vi "Coll_Det_Example.vi"() -> ()   [LabVIEW 2011]
uses:
  SObject.ctl
  Vector3D.ctl
panel:
  in  "Init Panel":T1={"Width"=800, "Lock to 60Hz?"=TRUE, "Height"=600, "Camera Type"=enum."Standard Camera", "Graphics Driver Type"=enum."DirectX 9"}
  in  "Probe Path Array":path[](array[path])=[path "cylinder.3DS"]
  in  "Moving Path Array":path[](array[path])=[path "cone.3DS", path "cylinder2.3DS"]
  in  "Static Path Array":path[](array[path])=[path "sphere.3DS", path "sphere2.3DS"]
  out "error out":errorcluster
  in  "stop":bool
  out "Collision Detected Array":bool[](array[boolean])
  in  "Moving Positions":T2
  out "FPS":i32=629
  out "SepDistance":T3[](array[typedef])=[{"X"=-12.215232849121094, "Y"=5.8577728271484375, "Z"=21.565397262573242}, {"X"=0.2394256591796875, "Y"=-15.688332557678223, "Z"=-24.610620498657227}, {"X"=126.86971282958984, "Y"=10.406116485595703, "Z"=28.3343563079834}, {"X"=-6.2993011474609375, "Y"=34.38507080078125, "Z"=60.643470764160156}]
  in  "Probe Position":T2
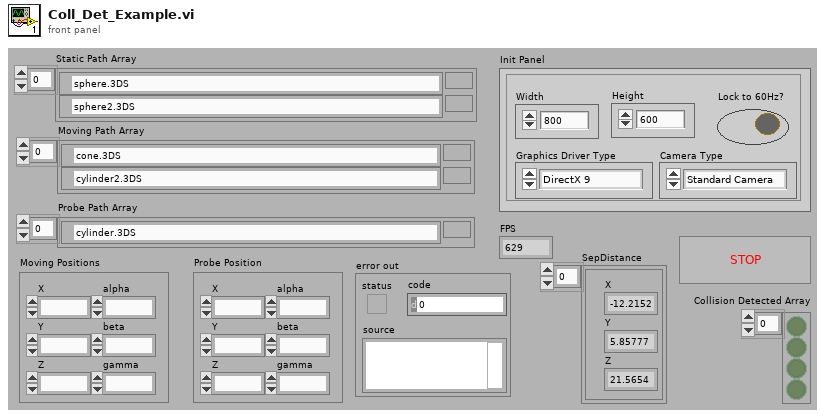
[diagram p1: front panel]
types:
  T1 = cluster{"Width":i32, "Lock to 60Hz?":bool, "Height":i32, "Camera Type":enum32{"Fixed Camera", "Standard Camera", "Flying Camera"}, "Graphics Driver Type":enum32{"No Driver (NULL)", "Software Driver", "Burnings Video", "DirectX 8", "DirectX 9", "OpenGL", "Count"}}
  T2 = typedef "SObject.ctl" = cluster{"X":dbl, "Y":dbl, "Z":dbl, "alpha":dbl, "beta":dbl, "gamma":dbl}
  T3 = typedef "Vector3D.ctl" = cluster{"X":dbl, "Y":dbl, "Z":dbl}
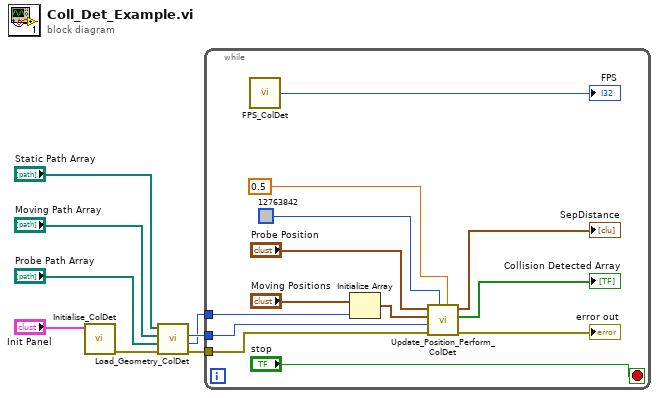
[diagram p0: block diagram]
diagram:
  n1 = call "Initialise_ColDet.vi"("Init Panel"="Init Panel") -> ("error out"=w8:errorcluster)  [unwired: 10 in]
  n2 = call "Load_Geometry_ColDet.vi"("error in"=w8, "Probe Path Array"="Probe Path Array", "Moving Path Array"="Moving Path Array", "Static Path Array"="Static Path Array") -> ("error out"=w7:errorcluster, "Number Moving"=w5:i32, "Number Static"=w6:i32)  [unwired: 5 in]
  n3 = while {
    tunnel: w7 -> [w21]
    tunnel: w5 -> [w15]
    tunnel: w6 -> [w20]
    stop <- "stop" stop-if-true
    n4 = call "FPS_ColDet.vi"() -> ("Current FPS"=→"FPS":i32)  [unwired: 6 in]
    n5 = Initialize Array("Moving Positions", w15) -> (w14:T2[])
    n6 = call "Update_Position_Perform_ColDet.vi"("Background Alpha"=0.5 ("Alpha"), "Background Color"=u32 12763842 ("Color"), "error in"=w21, "Number Static"=w20, "Moving Position Array"=w14, "Probe Position"="Probe Position") -> ("error out"=→"error out":errorcluster, "Collision Detected Array"=→"Collision Detected Array":bool[], "Separation Distance Array"=→"SepDistance":T3[])  [unwired: 3 in]
  }
